vi "Create 3D Projection.vi"(6 "Sub Object In":refnum<vi>, 7 "Projection Property":T3, 8 "error in (no error)":errorcluster, 9 "Actual Transform In":T1, 11 "Plot Object In":refnum<vi>) -> (0 "error out":errorcluster, 1 "Actual Transform Out":T1, 3 "Plot Object Out":refnum<vi>)   [LabVIEW 2020, in "3D Plot.lvclass"]
uses:
  <vilib>/Math Plots/3D Math Plots/3D Plot/3D Plot/3D Plot.lvclass
  <vilib>/Math Plots/3D Math Plots/3D Plot/3D Plot/Typedef/Actual Transform.ctl
  <vilib>/Math Plots/3D Math Plots/3D Plot/3D Plot/Typedef/Range Clusters.ctl
  <vilib>/picture/3D Picture Control/Object/Create Object (name).vi
  <vilib>/picture/3D Picture Control/NI_3D Picture Control.lvlib
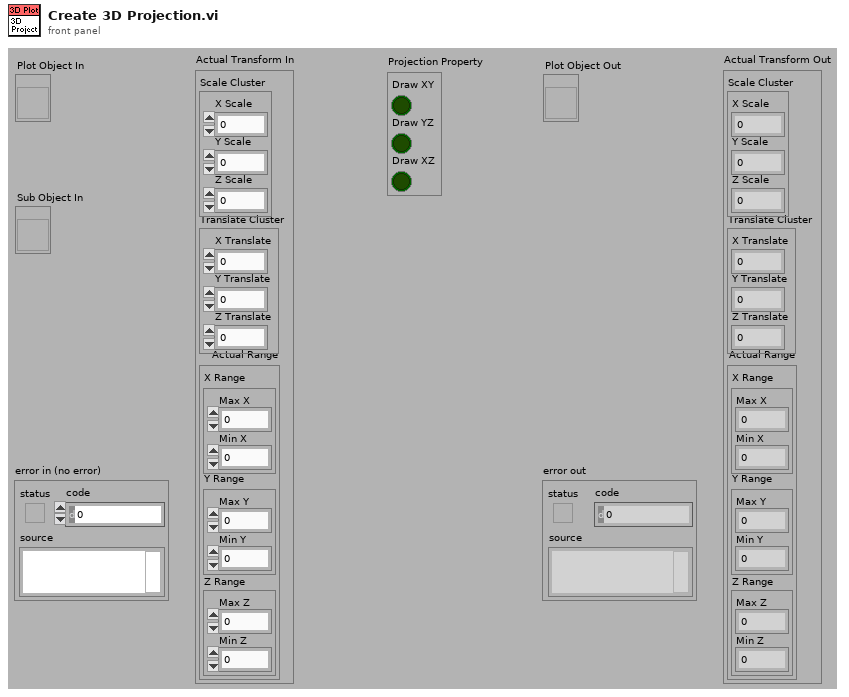
[diagram p1: front panel]
types:
  T1 = typedef "3D Plot.lvclass/Actual Transform.ctl" = cluster{"Scale Cluster":cluster{"X Scale":sgl, "Y Scale":sgl, "Z Scale":sgl}, "Translate Cluster":cluster{"X Translate":sgl, "Y Translate":sgl, "Z Translate":sgl}, "Actual Range":T2}
  T2 = typedef "3D Plot.lvclass/Range Clusters.ctl" = cluster{"X Range":cluster{"Max X":sgl, "Min X":sgl}, "Y Range":cluster{"Max Y":sgl, "Min Y":sgl}, "Z Range":cluster{"Max Z":sgl, "Min Z":sgl}}
  T3 = cluster{"Draw XY":bool, "Draw YZ":bool, "Draw XZ":bool}
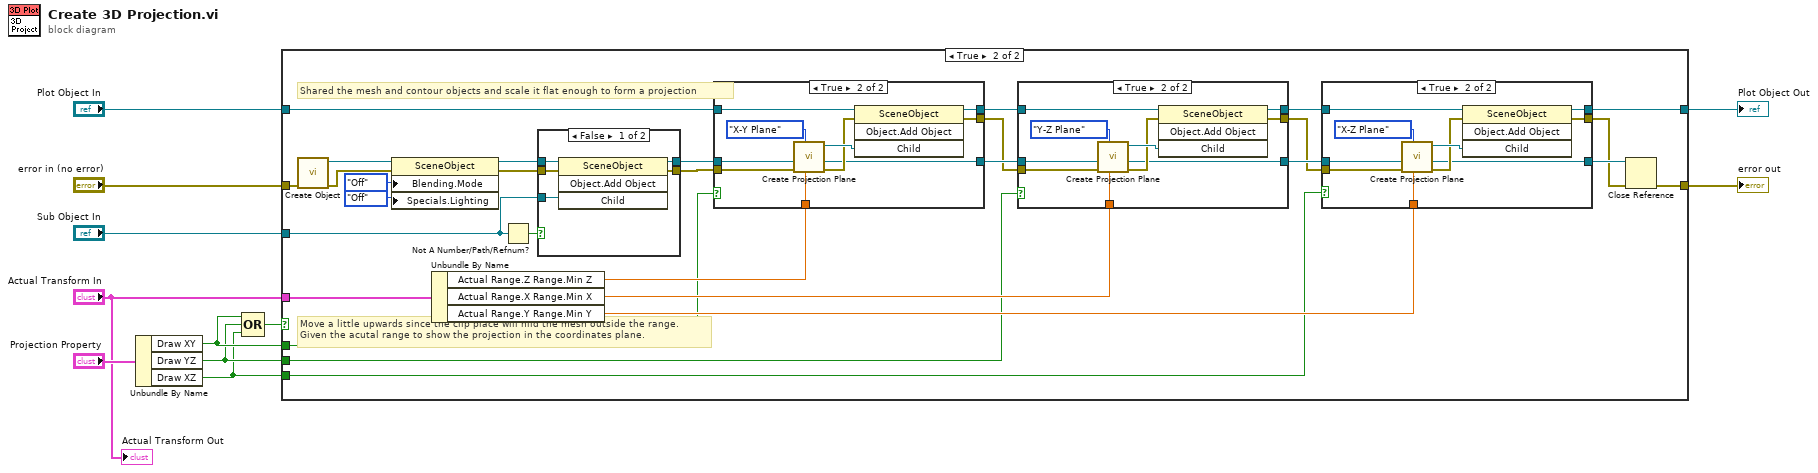
[diagram p0: block diagram]
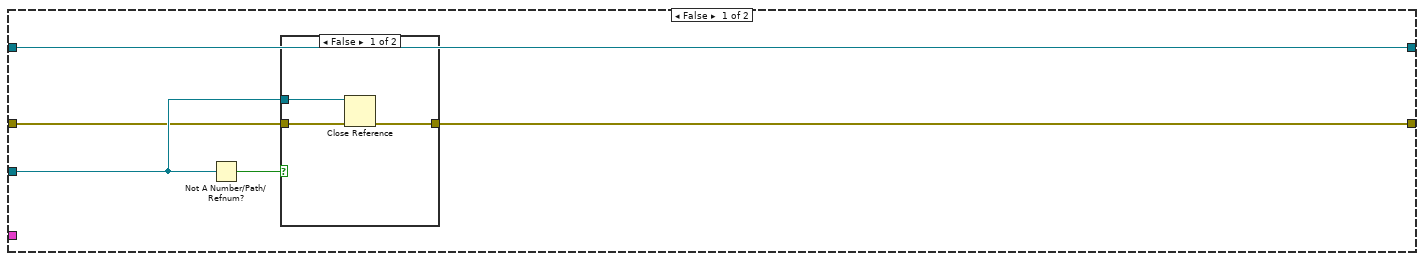
[diagram p2: hidden frame]
diagram:
  n1 = Unbundle By Name("Projection Property") -> ("Draw XY"=w4:bool, "Draw YZ"=w3:bool, "Draw XZ"=w2:bool)
  n2 = Compound Arithmetic op=OR(w4, w3, w2) -> (w1:bool)
  n3 = case shown="True" w1 {
    tunnel: "Plot Object In" -> [w16 w45]
    tunnel: [w16 w27] -> w9
    tunnel: "Sub Object In" -> [w14 w24]
    tunnel: "Actual Transform In" -> [_ w32]
    tunnel: "error in (no error)" -> [w13 w31]
    tunnel: [w12 w22] -> w5
    tunnel: w4 -> [_ w30]
    tunnel: w3 -> [_ w29]
    tunnel: w2 -> [_ w28]
    frame False {
      n4 = Not A Number/Path/Refnum?(number/path/refnum=w14) -> (NaN/Path/Refnum?=w15:bool)
      n5 = case shown="False" w15 {
        tunnel: w14 -> [w19 _]
        tunnel: w13 -> [w18 w20]
        tunnel: [w17 w20] -> w12
        frame False {
          n6 = Close Reference(reference=w19, error in (no error)=w18) -> (error out=w17:errorcluster)
        }
        frame True {
        }
      }
    }
    frame True {
      # "Shared the mesh and contour objects and scale it flat enough to form a projection"
      # "Move a little upwards since the clip place will hild the mesh outside the range.\nGiven the acutal range to show the projection in the coordinates plane."
      n7 = call-poly <vilib>:"Create Object.vi"("error in (no error)"=w31) -> ("error out"=w40:errorcluster, "Scene:New Object"=w46:refnum<vi>)  [unwired: 9 in]
      n8 = property class="SceneObject"(reference=w46, error in=w40, "Blending.Mode"=enum16{"Inherit Value", "Off", "On"}."Off" ("Blending:Mode"), "Specials.Lighting"=enum16{"Inherit Value", "Off", "On"}."Off" ("Specials:Lighting")) -> (reference out=w47:refnum<vi>, error out=w39:errorcluster)
      n9 = Unbundle By Name(w32) -> ("Actual Range.Z Range.Min Z"=w33:sgl, "Actual Range.X Range.Min X"=w34:sgl, "Actual Range.Y Range.Min Y"=w35:sgl)
      n10 = Not A Number/Path/Refnum?(number/path/refnum=w24) -> (NaN/Path/Refnum?=w36:bool)
      n11 = case shown="False" w36 {
        tunnel: w47 -> [w54 w56]
        tunnel: [w53 w56] -> w26
        tunnel: w39 -> [w52 w55]
        tunnel: [w51 w55] -> w25
        tunnel: w24 -> [w50 _]
        frame False {
          n12 = invoke class="SceneObject" method="Object.Add Object"(reference=w54, error in=w52, "Child"=w50) -> (reference out=w53:refnum<vi>, error out=w51:errorcluster)  [unwired: 1 in, 2 out]
        }
        frame True {
        }
      }
      n13 = case shown="True" w30 {
        tunnel: w26 -> [w84 w87]
        tunnel: w45 -> [w85 w95]
        tunnel: [w85 w94] -> w44
        tunnel: w33 -> [_ w88]
        tunnel: [w84 w86] -> w42
        tunnel: w25 -> [w83 w92]
        tunnel: [w83 w90] -> w38
        frame False {
        }
        frame True {
          n14 = call <vilib>:"Create Projection Plane.vi"("Min"=w88, "Plane"=enum16{"X-Y Plane", "Y-Z Plane", "X-Z Plane"}."X-Y Plane", "error out (no error)"=w92, "Origin Plot Ref"=w87) -> ("error out"=w91:errorcluster, "Dup Origin Plot Ref"=w86:refnum<vi>, "Projection Object Ref"=w93:refnum<vi>)  [unwired: 1 in, 4 out]
          n15 = invoke class="SceneObject" method="Object.Add Object"(reference=w95, error in=w91, "Child"=w93) -> (reference out=w94:refnum<vi>, error out=w90:errorcluster)  [unwired: 1 in, 2 out]
        }
      }
      n16 = case shown="True" w29 {
        tunnel: w44 -> [w72 w82]
        tunnel: [w72 w81] -> w43
        tunnel: w34 -> [_ w78]
        tunnel: w42 -> [w71 w74]
        tunnel: [w71 w73] -> w41
        tunnel: w38 -> [w70 w79]
        tunnel: [w70 w80] -> w37
        frame False {
        }
        frame True {
          n17 = call <vilib>:"Create Projection Plane.vi"("Min"=w78, "Plane"=enum16{"X-Y Plane", "Y-Z Plane", "X-Z Plane"}."Y-Z Plane", "error out (no error)"=w79, "Origin Plot Ref"=w74) -> ("error out"=w76:errorcluster, "Dup Origin Plot Ref"=w73:refnum<vi>, "Projection Object Ref"=w77:refnum<vi>)  [unwired: 1 in, 4 out]
          n18 = invoke class="SceneObject" method="Object.Add Object"(reference=w82, error in=w76, "Child"=w77) -> (reference out=w81:refnum<vi>, error out=w80:errorcluster)  [unwired: 1 in, 2 out]
        }
      }
      n19 = case shown="True" w28 {
        tunnel: w43 -> [w59 w69]
        tunnel: [w59 w68] -> w27
        tunnel: w35 -> [_ w62]
        tunnel: w41 -> [w58 w61]
        tunnel: w37 -> [w57 w66]
        tunnel: [w57 w67] -> w21
        tunnel: [w58 w60] -> w23
        frame False {
        }
        frame True {
          n20 = call <vilib>:"Create Projection Plane.vi"("Min"=w62, "Plane"=enum16{"X-Y Plane", "Y-Z Plane", "X-Z Plane"}."X-Z Plane", "error out (no error)"=w66, "Origin Plot Ref"=w61) -> ("error out"=w63:errorcluster, "Dup Origin Plot Ref"=w60:refnum<vi>, "Projection Object Ref"=w64:refnum<vi>)  [unwired: 1 in, 4 out]
          n21 = invoke class="SceneObject" method="Object.Add Object"(reference=w69, error in=w63, "Child"=w64) -> (reference out=w68:refnum<vi>, error out=w67:errorcluster)  [unwired: 1 in, 2 out]
        }
      }
      n22 = Close Reference(reference=w23, error in (no error)=w21) -> (error out=w22:errorcluster)
    }
  }
  "Plot Object Out" <- w9
  "error out" <- w5
  "Actual Transform Out" <- "Actual Transform In"
